vi "PatternGenMod_3.vi"(11 "DC offset":sgl) -> (3 "array":sgl[](array[numeric]))   [LabVIEW 2015]
uses:
  <vilib>/rvi/Emulation/niFpgaGetClockAttributes.vi
  <vilib>/rvi/Emulation/niFpgaSctlEmulationGetInTimedLoop.vi
  <vilib>/rvi/Emulation/niFpgaEmulationReportErrorSimple.vi
  <vilib>/rvi/Emulation/niFpgaCriticalErrorInLSC.vi
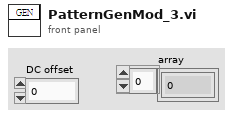
[diagram p1: front panel]
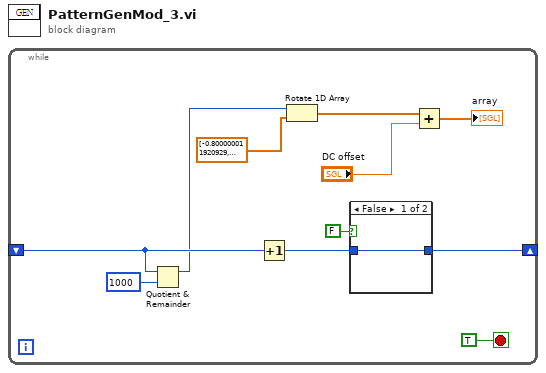
[diagram p0: block diagram]
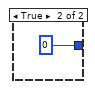
[diagram p2: hidden frame]
diagram:
  n1 = while {
    shift-right: [w6] -> _
    shift-left: _ -> [w9]
    stop <- TRUE stop-if-true
    n2 = Quotient & Remainder(x=w9, y=1000) -> (x-y*floor(x/y)=w4:i32)  [unwired: 1 out]
    n3 = Increment(x=w9) -> (x+1=w7:i32)
    n4 = Rotate 1D Array(1:sgl[] [-0.8, -0.75, -0.7, -0.65, -0.6, -0.55, -0.5, -0.45, -0.4, -0.35, -0.3, -0.25, -0.2, -0.15, -0.1, -0.05, 0.0, 0.05, 0.1, 0.15, 0.2, 0.25, 0.3, 0.35, 0.4, 0.45, 0.5, 0.55, 0.6, 0.65, 0.7, 0.75] ("x/y"), 2:w4) -> (0:w3:sgl[])
    n5 = case shown="False" FALSE {
      tunnel: w7 -> [w12 _]
      tunnel: [w12 0] -> w6
      frame False {
      }
      frame True {
      }
    }
    n6 = Add(x=w3, y="DC offset") -> (x+y=→"array":sgl[])
  }
